vi "SELECT FROM DB.vi"(8 "error in":errorcluster, 10 "object":refnum<class "_ISerializable.lvclass">, 11 "orm in":refnum<class "LV-ORM.lvclass">) -> (0 "error out":errorcluster, 1 "all obj":refnum<class "_ISerializable.lvclass">[](array[class]), 3 "orm out":refnum<class "LV-ORM.lvclass">, 4 "data":string[][](array[string]), 6 "column names":string[](array[string]))   [LabVIEW 2018, in "LV-ORM.lvclass"]
uses:
  LV-ORM.lvclass
  _Serializable Base Object/_ISerializable.lvclass
  Serializer/Serializer.lvclass
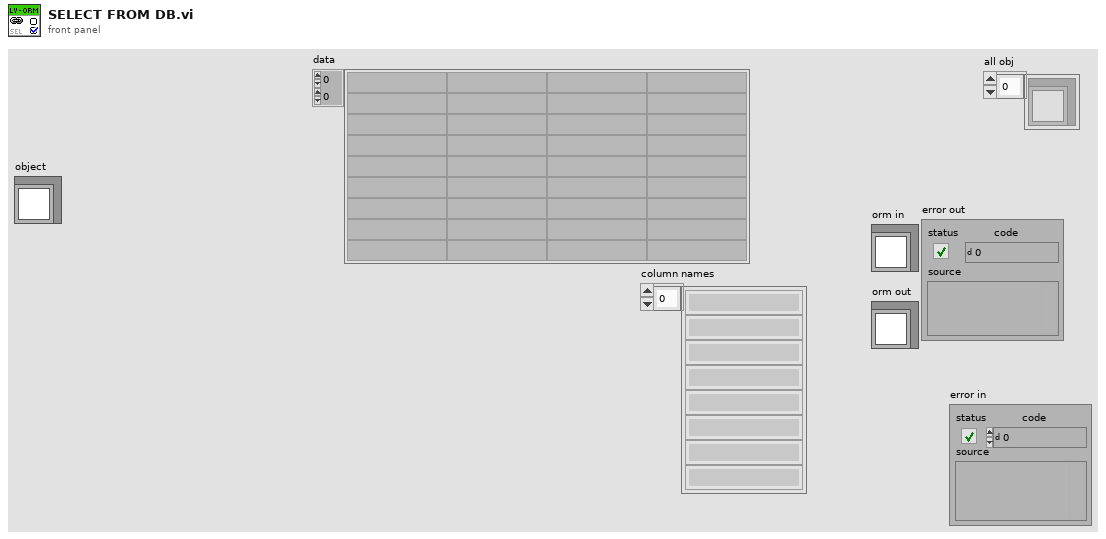
[diagram p1: front panel]
types:
  T1 = typedef "key-value-type cluster.ctl" = cluster{"names":string[], "values":string[], "type":string[], "class name":string}
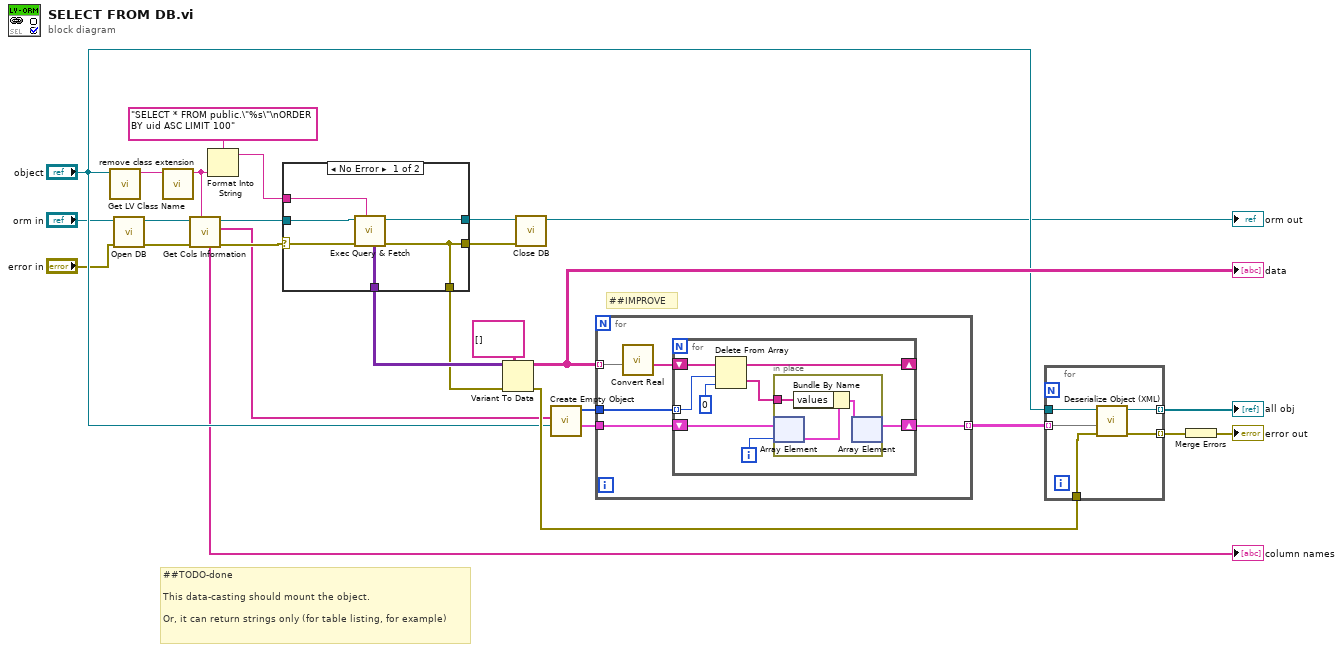
[diagram p0: block diagram]
diagram:
  # "##IMPROVE"
  # "##TODO-done\n\nThis data-casting should mount the object.\n\nOr, it can return strings only (for table listing, for example)"
  n1 = call <vilib>:"Get LV Class Name.vi"("object"="object") -> ("class name"=w27:string)  [unwired: 9 in, 1 out]
  n2 = call "Open DB.vi"("error in (no error)"="error in", "LV-ORM in"="orm in") -> ("error out"=w5:errorcluster, "LV-ORM out"=w6:refnum<class "LV-ORM.lvclass">)  [unwired: 8 in]
  n3 = call "remove class extension.vi"("class name in"=w27) -> ("class name out"=w14:string)  [unwired: 10 in]
  n4 = call "Get Cols Information.vi"("Table Name"=w14, "error in (no error)"=w5, "LV-ORM in"=w6) -> ("error out"=w15:errorcluster, "columns data type"=w10:string[], "LV-ORM out"=w16:refnum<class "LV-ORM.lvclass">, "column names"=→"column names":string[])  [unwired: 4 in, 1 out]
  n5 = Format Into String(format string="SELECT * FROM public.\"%s\"\nORDER BY uid ASC LIMIT 100", w14) -> (resulting string=w23:string)  [unwired: 2 in, 1 out]
  n6 = case shown="No Error" w15 {
    selector: w15 -> [w31 w34]
    tunnel: w16 -> [w30 w35]
    tunnel: [w33 _] -> w24
    tunnel: w23 -> [w32 _]
    tunnel: [w29 w35] -> w8
    tunnel: [w28 w34] -> w21
    tunnel: [w28 w34] -> w3
    frame No Error {
      n7 = call "Exec Query & Fetch.vi"("scripts"=w32, "error in"=w31, "orm in"=w30) -> ("error out"=w28:errorcluster, "orm out"=w29:refnum<class "LV-ORM.lvclass">, "recordset data"=w33:variant[][])  [unwired: 6 in]
    }
    frame Error {
    }
  }
  n8 = Variant To Data(error in=w21, type=string[][] [], Variant=w24) -> (data=w22:string[][], error out=w11:errorcluster)
  "data" <- w22
  n9 = call "Close DB.vi"("error in"=w3, "LV-ORM in"=w8) -> ("LV-ORM out"=→"orm out":refnum<class "LV-ORM.lvclass">)  [unwired: 8 in, 1 out]
  n10 = call "Create Empty Object.vi"("object"="object", "columns data type"=w10) -> ("Array 3"=w12:T1[], "elements by level"=w13:i32[])  [unwired: 8 in]
  n11 = for {
    tunnel: w22 -> [w37] mode=indexing
    tunnel: [w40] -> w20 mode=indexing
    tunnel: w13 -> [w39]
    tunnel: w12 -> [w38]
    n12 = call "Convert Real.vi"("data in"=w37) -> ("data out"=w36:string[])  [unwired: 10 in]
    n13 = for {
      shift-right: [w41] -> w40
      shift-left: w38 -> [w46]
      shift-right: [w43] -> _
      shift-left: w36 -> [w48]
      tunnel: w39 -> [w47] mode=indexing
      i -> [w45]
      n14 = Delete From Array(array=w48, length=w47, index=0) -> (deleted portion=w44:string[], array with subset deleted=w43:string[])
      n15 = in-place {
        in-place-border: w44 -> [w49]
        n16 = in-place-array #1(w46, w45) -> (w51:T1)
        n17 = Bundle By Name(cluster=w51, "values"=w49) -> (w50:T1)
        n18 = in-place-array #1(w50) -> (w41:T1[])  [unwired: 1 out]
      }
    }
  }
  n19 = for {
    tunnel: w20 -> [w54] mode=indexing
    tunnel: "object" -> [w56]
    tunnel: [w55] -> w19 mode=indexing
    tunnel: w11 -> [w53]
    tunnel: [w52] -> w18 mode=indexing
    n20 = call "Deserialize Object (XML).vi"("error in"=w53, "key-value-type in"=w54, "object type"=w56) -> ("casting error"=w52:errorcluster, "object out"=w55:refnum<class "_ISerializable.lvclass">)  [unwired: 7 in]
  }
  "all obj" <- w19
  n21 = Merge Errors(w18) -> (→"error out":errorcluster)
